vi "Get_Plugins_Available.vi"(11 "Reload Available Plugins":bool) -> (0 "Final":string[](array[string]), 1 "Per Block":string[](array[string]), 2 "Pre-Analysis":string[](array[string]), 3 "Initial":string[](array[string]), 5 "Directories":path[](array[path]))   [LabVIEW 2018]
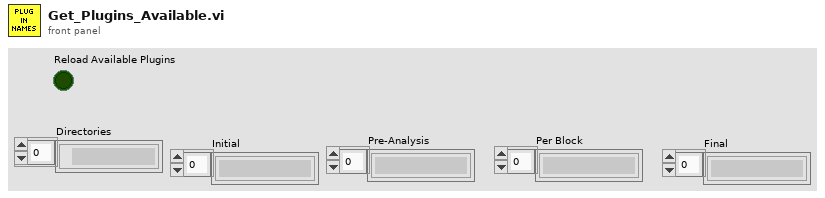
[diagram p1: front panel]
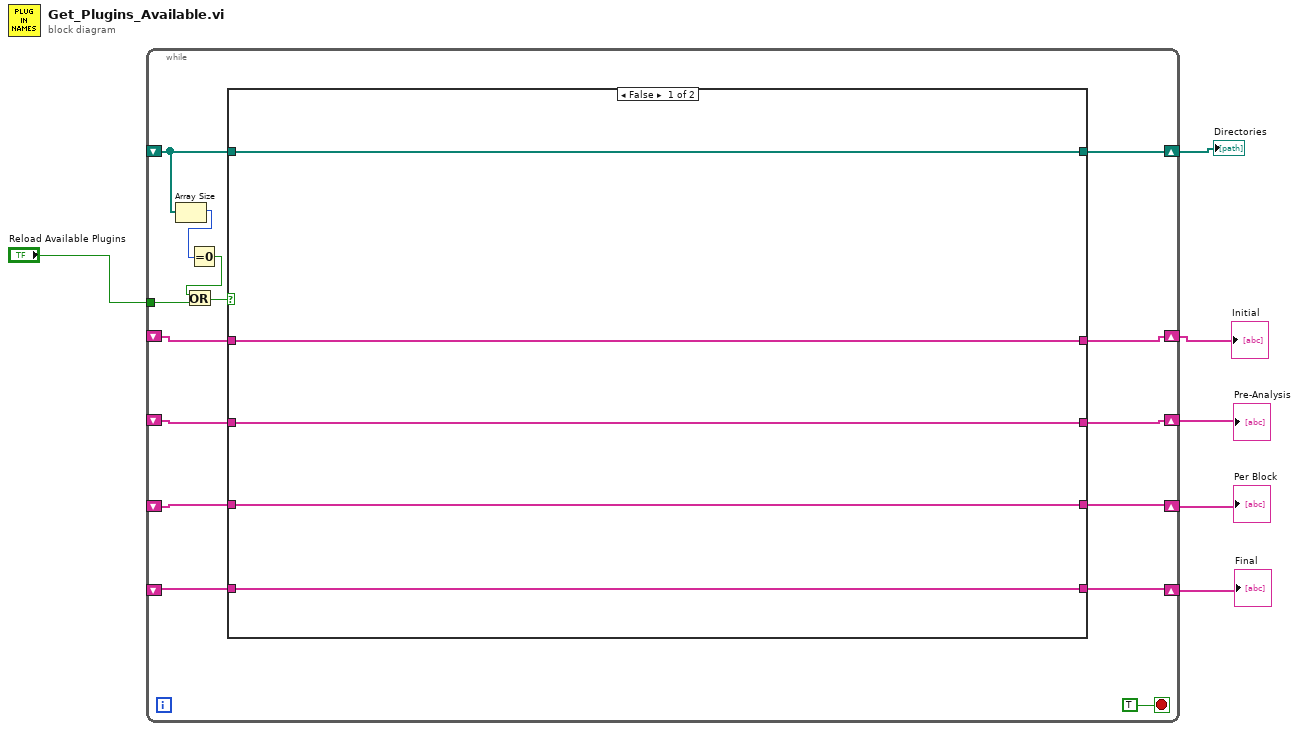
[diagram p0: block diagram]
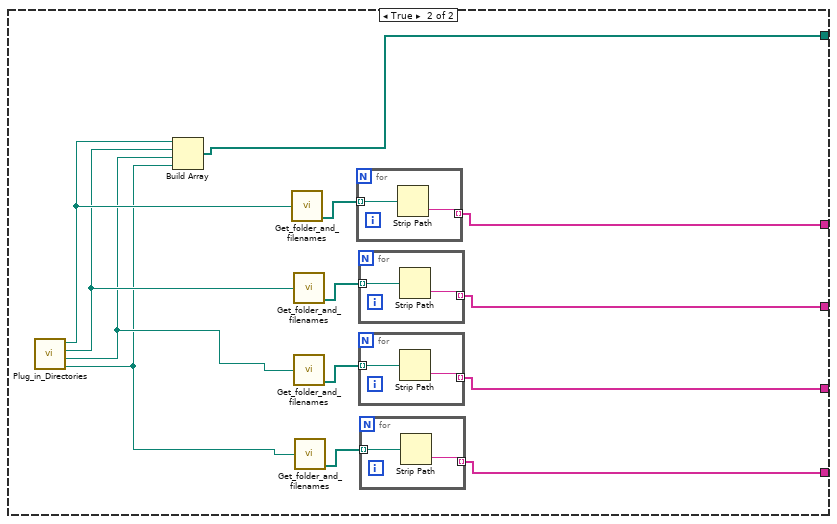
[diagram p2: hidden frame]
diagram:
  n1 = while {
    shift-right: [w21] -> w6
    shift-left: _ -> [w16]
    shift-right: [w20] -> w5
    shift-left: _ -> [w15]
    shift-right: [w19] -> w4
    shift-left: _ -> [w14]
    shift-right: [w18] -> w3
    shift-left: _ -> [w13]
    shift-right: [w17] -> w2
    shift-left: _ -> [w12]
    tunnel: "Reload Available Plugins" -> [w8]
    stop <- TRUE stop-if-true
    n2 = Array Size(array=w16) -> (size(s)=w10:i32)
    n3 = Equal To 0?(x=w10) -> (x = 0?=w9:bool)
    n4 = Or(x=w9, y=w8) -> (x .or. y?=w7:bool)
    n5 = case shown="False" w7 {
      tunnel: [w26 w38] -> w21
      tunnel: [w22 w30] -> w17
      tunnel: [w23 w29] -> w18
      tunnel: [w24 w28] -> w19
      tunnel: [w25 w27] -> w20
      tunnel: w16 -> [w26 _]
      tunnel: w15 -> [w25 _]
      tunnel: w14 -> [w24 _]
      tunnel: w13 -> [w23 _]
      tunnel: w12 -> [w22 _]
      frame False {
      }
      frame True {
        n6 = call "Plug_in_Directories.vi"() -> ("Initial"=w34:path, "Pre_Analysis_Plugins"=w33:path, "Per Block"=w32:path, "Final"=w31:path)  [unwired: 2 in, 1 out]
        n7 = Build Array(w34, w33, w32, w31) -> (w38:path[])
        n8 = call "Get_folder_and_filenames.vi"("file path (dialog if empty)"=w34) -> ("Files"=w39:path[])  [unwired: 1 out]
        n9 = call "Get_folder_and_filenames.vi"("file path (dialog if empty)"=w33) -> ("Files"=w37:path[])  [unwired: 1 out]
        n10 = call "Get_folder_and_filenames.vi"("file path (dialog if empty)"=w32) -> ("Files"=w36:path[])  [unwired: 1 out]
        n11 = call "Get_folder_and_filenames.vi"("file path (dialog if empty)"=w31) -> ("Files"=w35:path[])  [unwired: 1 out]
        n12 = for {
          tunnel: w39 -> [w47] mode=indexing
          tunnel: [w46] -> w27 mode=indexing
          n13 = Strip Path(path=w47) -> (name=w46:string)  [unwired: 1 out]
        }
        n14 = for {
          tunnel: w37 -> [w45] mode=indexing
          tunnel: [w44] -> w28 mode=indexing
          n15 = Strip Path(path=w45) -> (name=w44:string)  [unwired: 1 out]
        }
        n16 = for {
          tunnel: w36 -> [w43] mode=indexing
          tunnel: [w42] -> w29 mode=indexing
          n17 = Strip Path(path=w43) -> (name=w42:string)  [unwired: 1 out]
        }
        n18 = for {
          tunnel: w35 -> [w41] mode=indexing
          tunnel: [w40] -> w30 mode=indexing
          n19 = Strip Path(path=w41) -> (name=w40:string)  [unwired: 1 out]
        }
      }
    }
  }
  "Directories" <- w6
  "Initial" <- w5
  "Pre-Analysis" <- w4
  "Per Block" <- w3
  "Final" <- w2
